vi "ReadJSON.vi"(8 "error in (no error)":errorcluster) -> (0 "error out":errorcluster, 3 "JSON out":string)   [LabVIEW 2017, in "WebRead.lvlib"]
doc: "Read data from CoinDesk site.\nReturned in JSON format."
uses:
  WebRead.lvlib
  <vilib>/httpClient/LabVIEWHTTPClient.lvlib
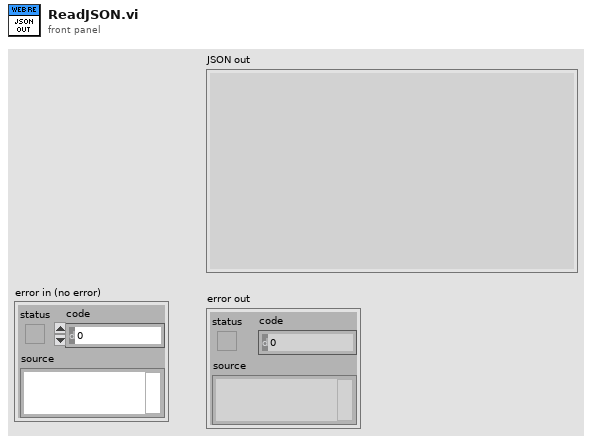
[diagram p1: front panel]
types:
  T1 = typedef "LabVIEWHTTPClient.lvlib/ClientHandle.ctl" = refnum<k1>
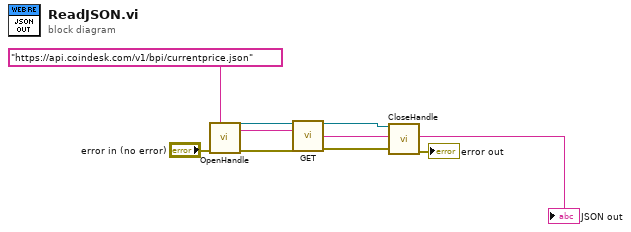
[diagram p0: block diagram]
diagram:
  n1 = call <vilib>:"OpenHandle.vi"("error in (no error)"="error in (no error)") -> ("client handle out"=w8:T1, "error out"=w4:errorcluster)  [unwired: 13 in]
  n2 = call <vilib>:"GET.vi"("client handle"=w8, "url"="https://api.coindesk.com/v1/bpi/currentprice.json", "error in (no error)"=w4) -> ("client handle out"=w7:T1, "body"=→"JSON out":string, "error out"=w3:errorcluster)  [unwired: 9 in, 1 out]
  n3 = call <vilib>:"CloseHandle.vi"("client handle"=w7, "error in (no error)"=w3) -> ("error out"=→"error out":errorcluster)  [unwired: 13 in]
